vi "Get All Simulated Addresses.vi"(8 "error in":errorcluster, 11 "Item Ref":T5 format="%.0x") -> (0 "error out":errorcluster, 2 "Simulated Addresses":T1[](array[typedef]) {"J1939 XNET Settings"."Name" format="%.0x"; "DM1 Data"."Data Reference" format="%.0x"; "DM1 Enable?"."Data Reference" format="%.0x"; "DM2 Data"."Data Reference" format="%.0x"; "DM2 Enable?"."Data Reference" format="%.0x"}, 3 "Item Ref out":T5 format="%.0x")   [LabVIEW 2013, in "J1939 Addon System Explorer.lvlib"]
uses:
  J1939 Addon System Explorer.lvlib
  <vilib>/NI Veristand/Custom Device API/Custom Device Item Ref.ctl
  Shared/Types/Compiled Simulated Settings.ctl
  Shared/Types/Monitor Settings.ctl
  <vilib>/NI Veristand/Custom Device API/Block Data Reference.ctl
  <vilib>/NI Veristand/Custom Device API/Data Reference.ctl
  <vilib>/NI Veristand/Custom Device API/Data Access Type.ctl
  <vilib>/NI Veristand/Custom Device Tools/Custom Device Utility Library/NI VeriStand - Search for All Items by GUID.vi
  Shared/SubVIs/Constants.vi
  <vilib>/NI Veristand/Custom Device API/Get Item Property (Variant).vi
  <vilib>/NI Veristand/Custom Device Tools/Custom Device Utility Library/Custom Device Utility Library.lvlib
  Shared/J1939 Addon Shared.lvlib
  <vilib>/NI Veristand/Custom Device API/Custom Device API.lvlib
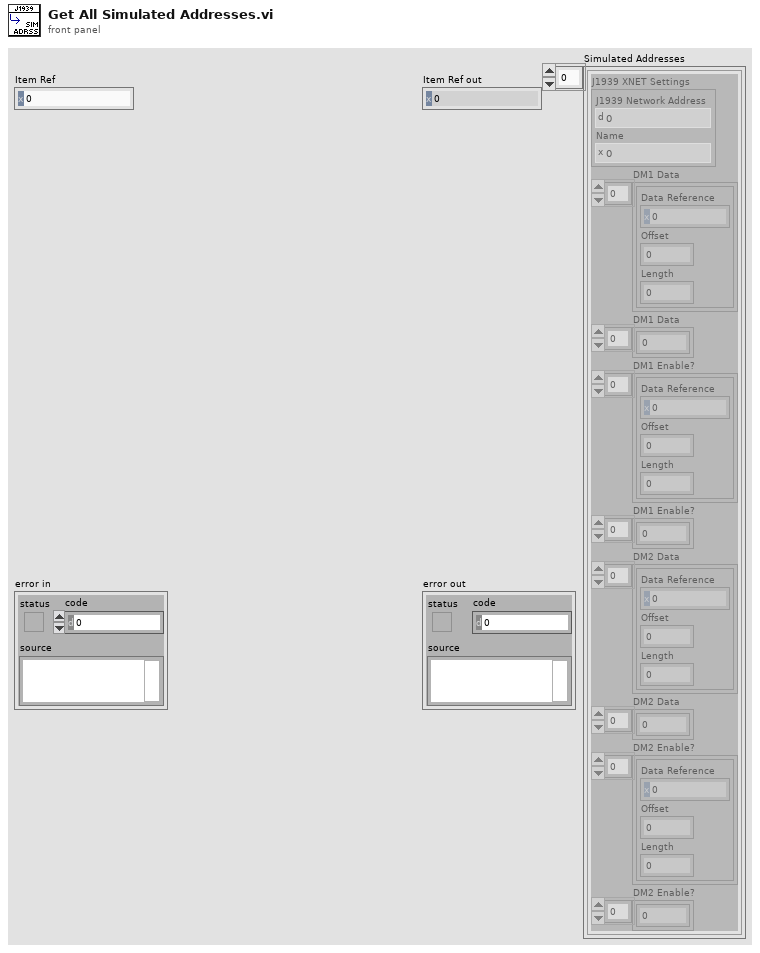
[diagram p1: front panel]
types:
  T1 = typedef "J1939 Addon Shared.lvlib/Compiled Simulated Settings.ctl" = cluster{"J1939 XNET Settings":T2, "DM1 Data":T3[], "DM1 Data":dbl[], "DM1 Enable?":T3[], "DM1 Enable?":dbl[], "DM2 Data":T3[], "DM2 Data":dbl[], "DM2 Enable?":T3[], "DM2 Enable?":dbl[]}
  T2 = typedef "J1939 Addon Shared.lvlib/Monitor Settings.ctl" = cluster{"J1939 Network Address":u8, "Name":u64}
  T3 = typedef "Custom Device API.lvlib/Block Data Reference.ctl" = cluster{"Data Reference":T4, "Offset":i32, "Length":i32}
  T4 = typedef "Custom Device API.lvlib/Data Reference.ctl" = i32
  T5 = typedef "Custom Device API.lvlib/Custom Device Item Ref.ctl" = u64
  T6 = typedef "Custom Device API.lvlib/Data Access Type.ctl" = enum16{"Read", "Write"}
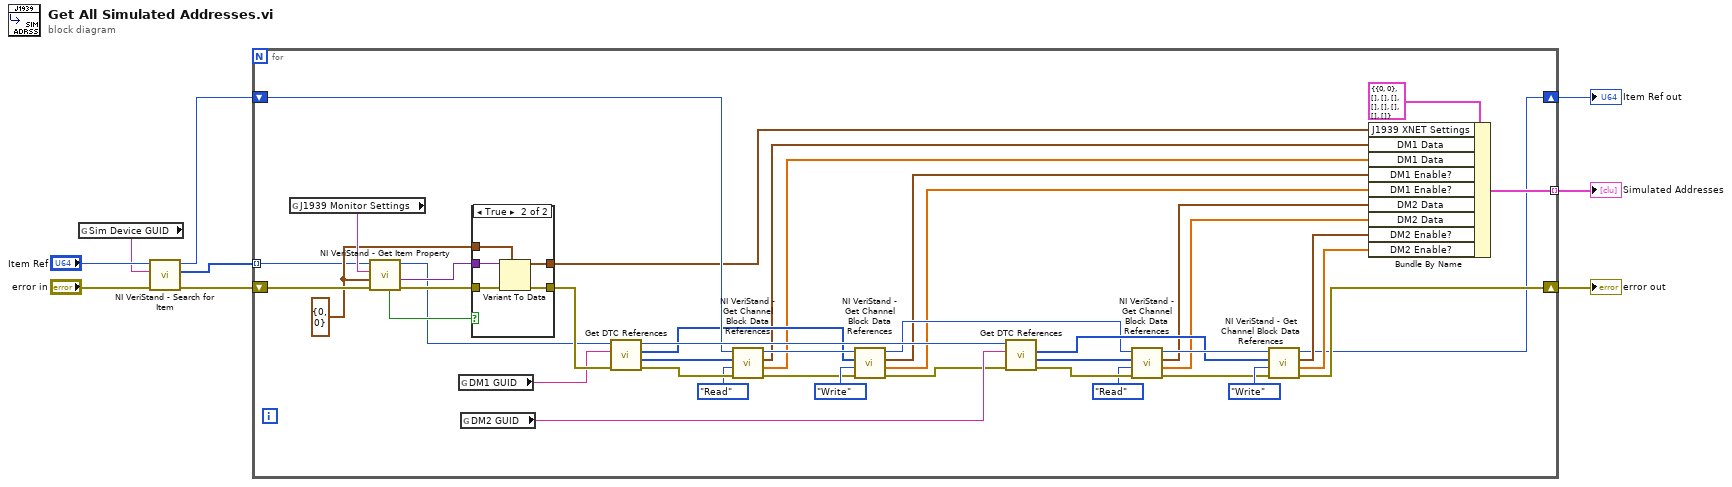
[diagram p0: block diagram]
diagram:
  n1 = global read "Constants.vi" "Sim Device GUID"() -> (w8:string)
  n2 = call-poly <vilib>:"NI VeriStand - Search for Item.vi"("error in"="error in", "Item GUID"=w8, "Section Ref in"="Item Ref") -> ("error out"=w7:errorcluster, "Item Refs"=w6:T5[], "Section Ref out"=w2:T5)  [unwired: 5 in, 1 out]
  n3 = for {
    shift-right: [w30] -> w4
    shift-left: w7 -> [w51]
    tunnel: w6 -> [w45] mode=indexing
    tunnel: [w12] -> w3 mode=indexing
    shift-right: [w10] -> w1
    shift-left: w2 -> [w37]
    w47 = T2 {"J1939 Network Address"=0, "Name"=0} ("J1939 XNET Settings")
    n4 = global read "Constants.vi" "J1939 Monitor Settings"() -> (w50:string)
    n5 = call-poly <vilib>:"NI VeriStand - Get Item Property.vi"("error in (no error)"=w51, "Default Value"=w47, "Property Name"=w50, "Item Ref in"=w45) -> ("error out"=w49:errorcluster, "Value"=w48:variant, "Item Ref out"=w43:T5, "Found?"=w46:bool)  [unwired: 4 in]
    n6 = global read "Constants.vi" "DM1 GUID"() -> (w42:string)
    n7 = global read "Constants.vi" "DM2 GUID"() -> (w41:string)
    n8 = case shown="True" w46 {
      tunnel: w49 -> [w52 w58]
      tunnel: w48 -> [_ w57]
      tunnel: w47 -> [w53 w56]
      tunnel: [w52 w55] -> w44
      tunnel: [w53 w54] -> w11
      frame False {
      }
      frame True {
        n9 = Variant To Data(error in=w58, type=w56, Variant=w57) -> (data=w54:T2, error out=w55:errorcluster)
      }
    }
    n10 = call "Get DTC References.vi"("error in (no error)"=w44, "DM GUID"=w42, "Item Ref in"=w43) -> ("error out"=w39:errorcluster, "Data"=w38:T5[], "Active"=w22:T5[], "Section Ref out"=w40:T5)  [unwired: 5 in]
    n11 = call <vilib>:"NI VeriStand - Get Channel Block Data References.vi"("error in (no error)"=w39, "Access"=Data_Access_Type."Read", "Channel Refs"=w38, "Device Ref in"=w37) -> ("error out"=w26:errorcluster, "Values Array"=w19:dbl[], "Block Data Refs"=w20:T3[], "Device Ref out"=w24:T5)  [unwired: 4 in]
    n12 = call <vilib>:"NI VeriStand - Get Channel Block Data References.vi"("error in (no error)"=w26, "Access"=Data_Access_Type."Write", "Channel Refs"=w22, "Device Ref in"=w24) -> ("error out"=w25:errorcluster, "Values Array"=w14:dbl[], "Block Data Refs"=w13:T3[], "Device Ref out"=w23:T5)  [unwired: 4 in]
    n13 = call "Get DTC References.vi"("error in (no error)"=w25, "DM GUID"=w41, "Item Ref in"=w40) -> ("error out"=w36:errorcluster, "Data"=w35:T5[], "Active"=w28:T5[])  [unwired: 5 in, 1 out]
    n14 = call <vilib>:"NI VeriStand - Get Channel Block Data References.vi"("error in (no error)"=w36, "Access"=Data_Access_Type."Read", "Channel Refs"=w35, "Device Ref in"=w23) -> ("error out"=w31:errorcluster, "Values Array"=w16:dbl[], "Block Data Refs"=w15:T3[], "Device Ref out"=w29:T5)  [unwired: 4 in]
    n15 = call <vilib>:"NI VeriStand - Get Channel Block Data References.vi"("error in (no error)"=w31, "Access"=Data_Access_Type."Write", "Channel Refs"=w28, "Device Ref in"=w29) -> ("error out"=w30:errorcluster, "Values Array"=w18:dbl[], "Block Data Refs"=w17:T3[], "Device Ref out"=w10:T5)  [unwired: 4 in]
    n16 = Bundle By Name(cluster=T1 {"J1939 XNET Settings"={"J1939 Network Address"=0, "Name"=0}, "DM1 Data"=[], "DM1 Data"=[], "DM1 Enable?"=[], "DM1 Enable?"=[], "DM2 Data"=[], "DM2 Data"=[], "DM2 Enable?"=[], "DM2 Enable?"=[]}, "J1939 XNET Settings"=w11, "DM1 Data"=w20, "DM1 Data"=w19, "DM1 Enable?"=w13, "DM1 Enable?"=w14, "DM2 Data"=w15, "DM2 Data"=w16, "DM2 Enable?"=w17, "DM2 Enable?"=w18) -> (w12:T1)
  }
  "error out" <- w4
  "Item Ref out" <- w1
  "Simulated Addresses" <- w3
